vi "Get PRL Command Queue.vi"(8 "error in (no error)":errorcluster) -> (0 "error out":errorcluster, 3 "PRL Command Queue":refnum<queue>)   [LabVIEW 2013, in "PMU Recorder Light.lvlib"]
uses:
  PMU Recorder Light.lvlib
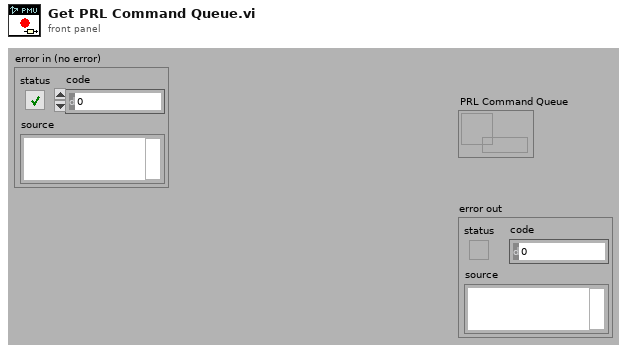
[diagram p1: front panel]
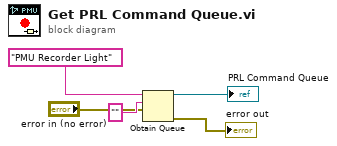
[diagram p0: block diagram]
diagram:
  n1 = Obtain Queue(name (unnamed)="PMU Recorder Light", element data type="" ("name (unnamed)"), error in (no error)="error in (no error)") -> (queue out=→"PRL Command Queue":refnum<queue>, error out=→"error out":errorcluster)  [unwired: 2 in, 1 out]
